vi "clear_fifos.vi"   [LabVIEW 2015]
uses:
  <vilib>/rvi/Emulation/niFpgaEmulationIsFPGAContextNoSignature.vi
  <vilib>/rvi/FIFO/Fifo_Resource/nirvififoEmulationSetSize.vi
  <vilib>/rvi/DataTransferAndStorage/Container/Common/niFpgaContainerGetUniqueNameForEmu.vi
  <vilib>/rvi/FIFO/Fifo_Resource/nirviFifoEmulationQueueMgr.vi
  <instcachedir>/0/nirviFifoEmulationQueueMgr_E5CAEC123FF24DC58D834DCA3CDAA9B5.lvgen/nirviFifoEmulationQueueMgr_E5CAEC123FF24DC58D834DCA3CDAA9B5_002.vi
  <vilib>/rvi/Emulation/niFpgaProcessEmulError.vi
  <instcachedir>/0/nirviFifoEmulationQueueMgr_E5CAEC123FF24DC58D834DCA3CDAA9B5.lvgen/nirviFifoEmulationQueueMgr_E5CAEC123FF24DC58D834DCA3CDAA9B5_001.vi
  <vilib>/rvi/DataTransferAndStorage/Container/XNode/niFpgaContainer.xnode
  <vilib>/rvi/FIFO/Fifo_Resource/nirvififoEmulationClear.vi
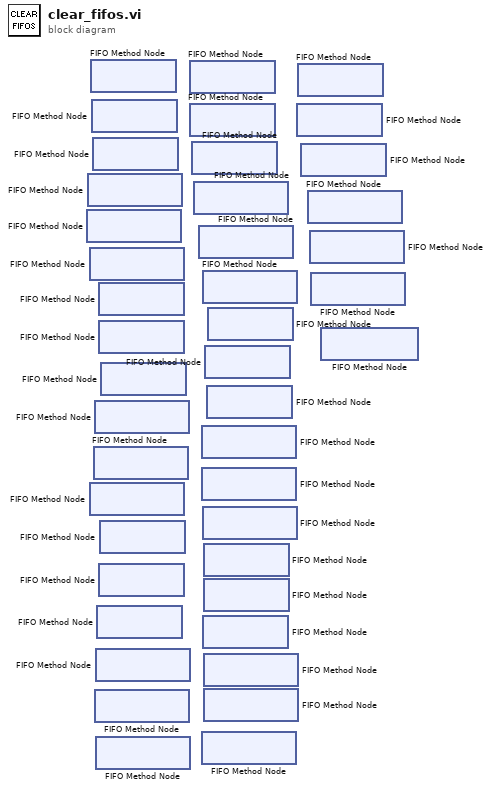
[diagram p0: block diagram]
diagram:
  n1 = xnode ("FIFO Method Node")() -> ()  [unwired: 1 in, 1 out]
  n2 = xnode ("FIFO Method Node")() -> ()  [unwired: 1 in, 1 out]
  n3 = xnode ("FIFO Method Node")() -> ()  [unwired: 1 in, 1 out]
  n4 = xnode ("FIFO Method Node")() -> ()  [unwired: 1 in, 1 out]
  n5 = xnode ("FIFO Method Node")() -> ()  [unwired: 1 in, 1 out]
  n6 = xnode ("FIFO Method Node")() -> ()  [unwired: 1 in, 1 out]
  n7 = xnode ("FIFO Method Node")() -> ()  [unwired: 1 in, 1 out]
  n8 = xnode ("FIFO Method Node")() -> ()  [unwired: 1 in, 1 out]
  n9 = xnode ("FIFO Method Node")() -> ()  [unwired: 1 in, 1 out]
  n10 = xnode ("FIFO Method Node")() -> ()  [unwired: 1 in, 1 out]
  n11 = xnode ("FIFO Method Node")() -> ()  [unwired: 1 in, 1 out]
  n12 = xnode ("FIFO Method Node")() -> ()  [unwired: 1 in, 1 out]
  n13 = xnode ("FIFO Method Node")() -> ()  [unwired: 1 in, 1 out]
  n14 = xnode ("FIFO Method Node")() -> ()  [unwired: 1 in, 1 out]
  n15 = xnode ("FIFO Method Node")() -> ()  [unwired: 1 in, 1 out]
  n16 = xnode ("FIFO Method Node")() -> ()  [unwired: 1 in, 1 out]
  n17 = xnode ("FIFO Method Node")() -> ()  [unwired: 1 in, 1 out]
  n18 = xnode ("FIFO Method Node")() -> ()  [unwired: 1 in, 1 out]
  n19 = xnode ("FIFO Method Node")() -> ()  [unwired: 1 in, 1 out]
  n20 = xnode ("FIFO Method Node")() -> ()  [unwired: 1 in, 1 out]
  n21 = xnode ("FIFO Method Node")() -> ()  [unwired: 1 in, 1 out]
  n22 = xnode ("FIFO Method Node")() -> ()  [unwired: 1 in, 1 out]
  n23 = xnode ("FIFO Method Node")() -> ()  [unwired: 1 in, 1 out]
  n24 = xnode ("FIFO Method Node")() -> ()  [unwired: 1 in, 1 out]
  n25 = xnode ("FIFO Method Node")() -> ()  [unwired: 1 in, 1 out]
  n26 = xnode ("FIFO Method Node")() -> ()  [unwired: 1 in, 1 out]
  n27 = xnode ("FIFO Method Node")() -> ()  [unwired: 1 in, 1 out]
  n28 = xnode ("FIFO Method Node")() -> ()  [unwired: 1 in, 1 out]
  n29 = xnode ("FIFO Method Node")() -> ()  [unwired: 1 in, 1 out]
  n30 = xnode ("FIFO Method Node")() -> ()  [unwired: 1 in, 1 out]
  n31 = xnode ("FIFO Method Node")() -> ()  [unwired: 1 in, 1 out]
  n32 = xnode ("FIFO Method Node")() -> ()  [unwired: 1 in, 1 out]
  n33 = xnode ("FIFO Method Node")() -> ()  [unwired: 1 in, 1 out]
  n34 = xnode ("FIFO Method Node")() -> ()  [unwired: 1 in, 1 out]
  n35 = xnode ("FIFO Method Node")() -> ()  [unwired: 1 in, 1 out]
  n36 = xnode ("FIFO Method Node")() -> ()  [unwired: 1 in, 1 out]
  n37 = xnode ("FIFO Method Node")() -> ()  [unwired: 1 in, 1 out]
  n38 = xnode ("FIFO Method Node")() -> ()  [unwired: 1 in, 1 out]
  n39 = xnode ("FIFO Method Node")() -> ()  [unwired: 1 in, 1 out]
  n40 = xnode ("FIFO Method Node")() -> ()  [unwired: 1 in, 1 out]
  n41 = xnode ("FIFO Method Node")() -> ()  [unwired: 1 in, 1 out]
  n42 = xnode ("FIFO Method Node")() -> ()  [unwired: 1 in, 1 out]
  n43 = xnode ("FIFO Method Node")() -> ()  [unwired: 1 in, 1 out]
